vi "RT DAQ.vi"() -> ()   [LabVIEW 2023]
uses:
  <vilib>/rvi/interface/nirviOpenFPGA/nirviOpenFPGA.xnode
  <vilib>/rvi/interface/nirviMethod/nirviMethod.xnode
  <vilib>/FPGAPlugInAG/Dynamic/niLvFpga_Run_Dynamic.vi
  <vilib>/rvi/interface/nirviMethod/StockFPGA_InlinedMethodWaitForSingleIRQ.vi
  <vilib>/FPGAPlugInAG/Dynamic/niLvFpga_WaitOnIrq_Dynamic.vi
  <vilib>/FPGAPlugInAG/Dynamic/niLvFpga_AcknowledgeIrq_Dynamic.vi
  <vilib>/FPGAPlugInAG/Dynamic/niLvFpga_Reset_Dynamic.vi
  <vilib>/rvi/interface/nirviReadWriteControl/nirviReadWriteControl.xnode
  NiFpgaLv.dll
  <vilib>/Utility/error.llb/Error Cluster From Error Code.vi
  <vilib>/rvi/interface/Simulation/niFpgaSimulationCallBeginRW.vi
  <vilib>/rvi/errors/niLvFpgaAdjustHostInterfaceError.vi
  <vilib>/rvi/interface/nirviCloseFPGA/nirviCloseFPGA.xnode
  <vilib>/NI_Real-Time Target Support.lvlib
  <vilib>/FPGAPlugInAG/Dynamic/niLvFpga_Close_Dynamic.vi
  Transport measurement/FPGA Bitfiles/Mainproject_FPGATarget_SinglepointDAQ2_KFK63D1NkjA.lvbitx
  Single point DAQ.vi
  <vilib>/FPGAPlugInAG/cRIO-9063/niLvFpga_Open_cRIO-9063.vi
  <vilib>/rvi/interface/common/dynamic/niFpgaDynamicAddResources.vi
panel:
  out "VI Stop":bool
  out "error out":errorcluster
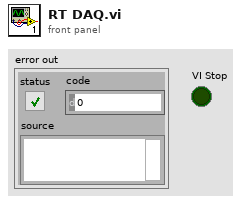
[diagram p1: front panel]
types:
  T1 = cluster{"Command":string, "Voltage":dbl, "Channel":string}
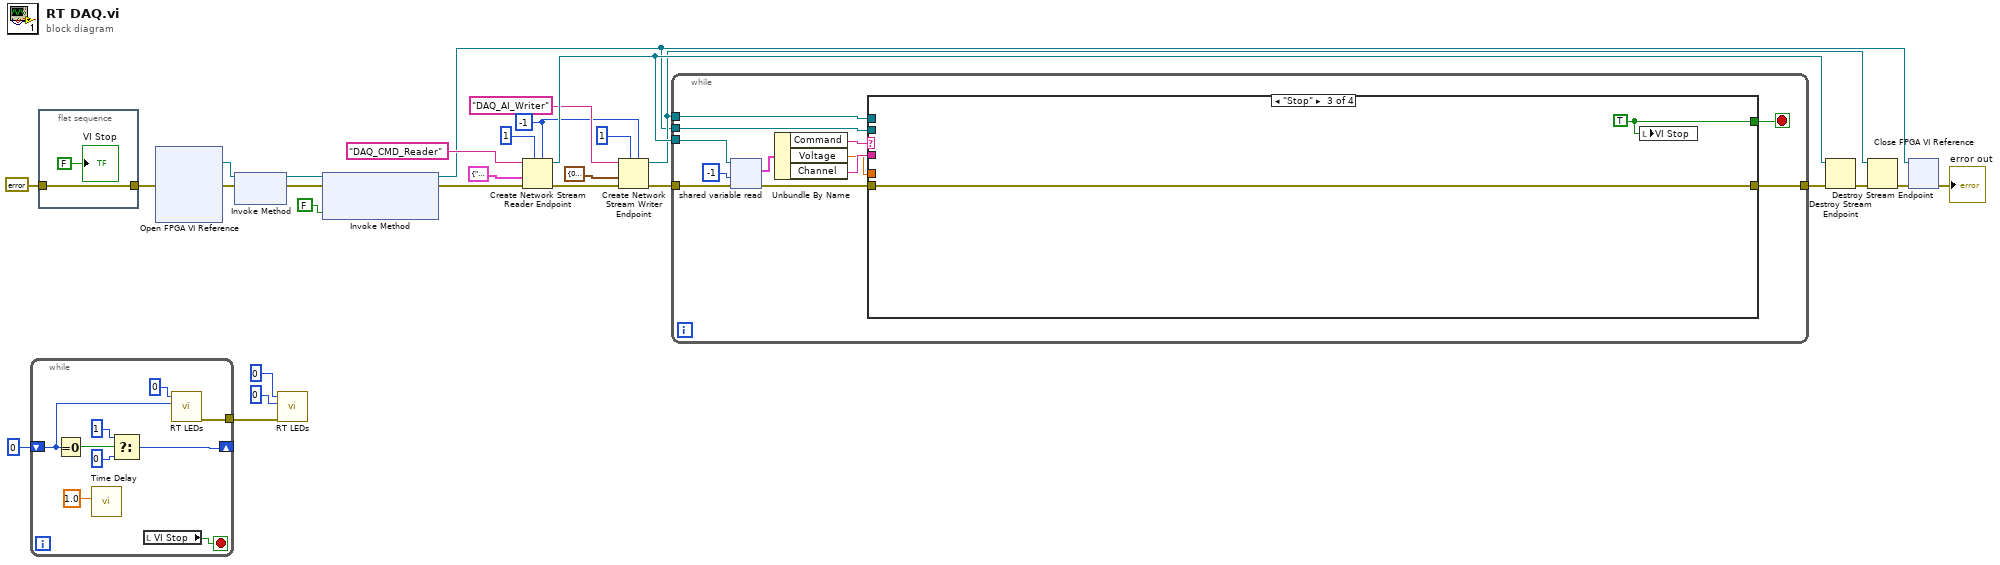
[diagram p0: block diagram]
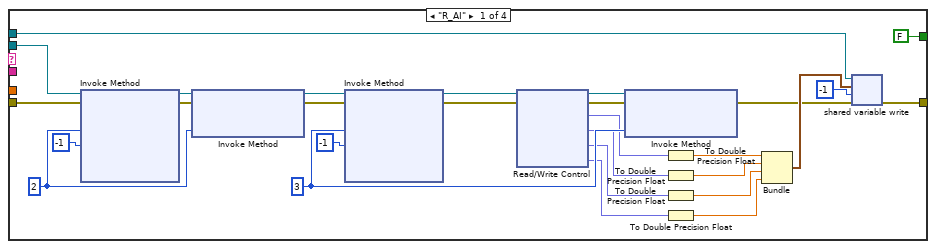
[diagram p2: hidden frame]
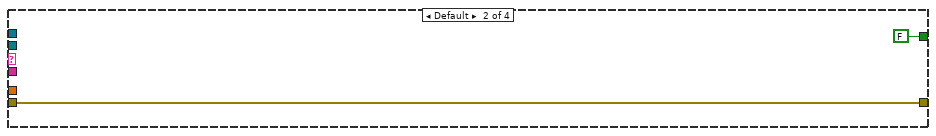
[diagram p3: hidden frame]
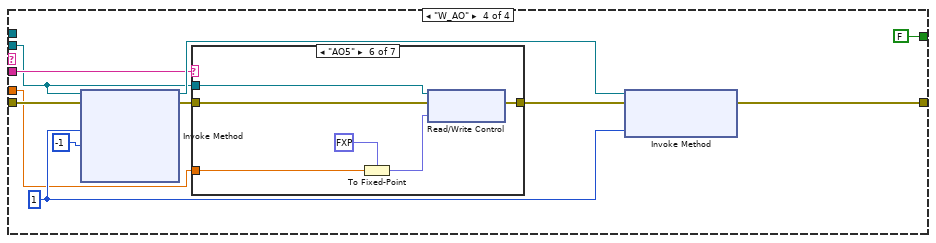
[diagram p4: hidden frame]
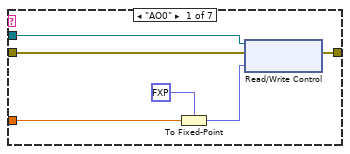
[diagram p5: hidden frame]
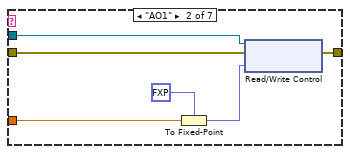
[diagram p6: hidden frame]
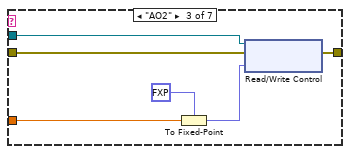
[diagram p7: hidden frame]
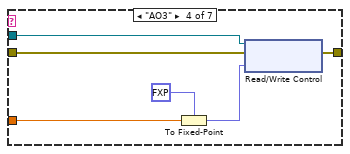
[diagram p8: hidden frame]
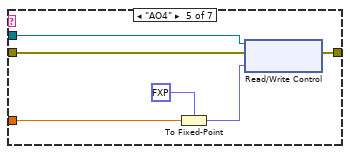
[diagram p9: hidden frame]
diagram:
  w1 = -1 ("timeout in ms (-1)")
  n1 = while {
    shift-right: [w32] -> _
    shift-left: 0 ("State") -> [w36]
    tunnel: [w29] -> w4
    stop <- w30 stop-if-true
    n2 = Equal To 0?(x=w36) -> (x = 0?=w35:bool)
    n3 = call "Time Delay"("Delay Time (s)"=1.0) -> ()  [unwired: 10 in, 1 out]
    n4 = Select(t=1, s=w35, f=0) -> (s? t:f=w32:i32)
    n5 = local read "VI Stop"() -> (w30:bool)
    n6 = call <vilib>:"RT LEDs.vi"("State"=w36, "LED Num"=0) -> ("error out"=w29:errorcluster)  [unwired: 4 in, 1 out]
  }
  n7 = flat-sequence {
    tunnel: errorcluster {"status"=FALSE, "code"=0, "source"=""} ("error in (no error)") -> [w39]
    tunnel: [w39] -> w2
    frame #0 {
      "VI Stop" <- FALSE ("VI Stop")
    }
  }
  n8 = xnode "Open FPGA VI Reference"("error in"=w2) -> ("FPGA VI Reference Out"=w24:refnum<k20>, "error out"=w23:errorcluster)  [unwired: 1 in]
  n9 = xnode "Invoke Method"("FPGA VI Reference In"=w24, "error in"=w23) -> ("FPGA VI Reference Out"=w25:refnum<k20>, "error out"=w22:errorcluster)
  n10 = call <vilib>:"RT LEDs.vi"("error in (no error)"=w4, "State"=0, "LED Num"=0) -> ()  [unwired: 3 in, 2 out]
  n11 = xnode "Invoke Method"("FPGA VI Reference In"=w25, "error in"=w22, "Wait Until Done (F)"=FALSE) -> ("FPGA VI Reference Out"=w11:refnum<k20>, "error out"=w17:errorcluster)
  n12 = Create Network Stream Reader Endpoint(5:w1, 7:1 ("reader buffer size"), 8:w17, 9:T1 {"Command"="", "Voltage"=0.0, "Channel"=""} ("Write cluster"), 11:"DAQ_CMD_Reader" ("reader name")) -> (0:w14:errorcluster, 3:w20:refnum<k21>)  [unwired: 2 in]
  n13 = Create Network Stream Writer Endpoint(5:w1, 7:1 ("writer buffer size"), 8:w14, 9:cluster{dbl, dbl, dbl, dbl} {0.0, 0.0, 0.0, 0.0} ("output cluster"), 11:"DAQ_AI_Writer" ("reader name")) -> (0:w9:errorcluster, 3:w13:refnum<k21>)  [unwired: 2 in]
  n14 = while {
    tunnel: w9 -> [w51]
    tunnel: w20 -> [w50]
    tunnel: w11 -> [w46]
    tunnel: [w41] -> w21
    tunnel: w13 -> [w42]
    stop <- w40 stop-if-true
    n15 = shared-variable-read(w50, w51, -1 ("timeout ms (-1)")) -> (w45:errorcluster, w48:T1)  [unwired: 2 out]
    n16 = Unbundle By Name(w48) -> ("Command"=w47:string, "Voltage"=w43:dbl, "Channel"=w44:string)
    n17 = case shown="\"Stop\"" w47 {
      tunnel: w46 -> [w74 _ _ w87]
      tunnel: w45 -> [w75 w80 w83 w90]
      tunnel: w44 -> [_ _ _ w88]
      tunnel: w43 -> [_ _ _ w86]
      tunnel: [w53 w80 w83 w85] -> w41
      tunnel: w42 -> [w65 _ _ _]
      tunnel: [FALSE FALSE w82 FALSE] -> w40
      frame "R_AI" {
        w73 = 3 ("IRQ Number(s)")
        w77 = 2 ("IRQ Number(s)")
        n18 = xnode "Invoke Method"("FPGA VI Reference In"=w74, "error in"=w75, "IRQ Number(s)"=w77, "Timeout (ms)"=-1) -> ("FPGA VI Reference Out"=w78:refnum<k20>, "error out"=w79:errorcluster)  [unwired: 2 out]
        n19 = xnode "Invoke Method"("FPGA VI Reference In"=w78, "error in"=w79, "IRQ Number(s)"=w77) -> ("FPGA VI Reference Out"=w71:refnum<k20>, "error out"=w70:errorcluster)
        n20 = xnode "Invoke Method"("FPGA VI Reference In"=w71, "error in"=w70, "IRQ Number(s)"=w73, "Timeout (ms)"=-1) -> ("FPGA VI Reference Out"=w69:refnum<k20>, "error out"=w68:errorcluster)  [unwired: 2 out]
        n21 = xnode "Read/Write Control"("FPGA VI Reference In"=w69, "error in"=w68) -> ("FPGA VI Reference Out"=w67:refnum<k20>, "error out"=w66:errorcluster, "Mod1/AI0"=w64:fxp<+/-,17,5>, "Mod1/AI1"=w63:fxp<+/-,17,5>, "Mod1/AI2"=w62:fxp<+/-,17,5>, "Mod1/AI3"=w61:fxp<+/-,17,5>)
        n22 = xnode "Invoke Method"("FPGA VI Reference In"=w67, "error in"=w66, "IRQ Number(s)"=w73) -> ("error out"=w55:errorcluster)  [unwired: 1 out]
        n23 = To Double Precision Float(number=w64) -> (double precision float=w60:dbl)
        n24 = To Double Precision Float(number=w63) -> (double precision float=w59:dbl)
        n25 = To Double Precision Float(number=w62) -> (double precision float=w58:dbl)
        n26 = To Double Precision Float(number=w61) -> (double precision float=w57:dbl)
        n27 = Bundle(w60, w59, w58, w57) -> (w56:cluster{dbl, dbl, dbl, dbl})  [unwired: 1 in]
        n28 = shared-variable-write(w65, w55, w56, -1 ("timeout ms (-1)")) -> (w53:errorcluster)  [unwired: 2 out]
      }
      frame Default {
      }
      frame "Stop" {
        w82 = TRUE
        n29 = local write "VI Stop"(w82) -> ()
      }
      frame "W_AO" {
        w91 = 1 ("IRQ Number(s)")
        n30 = xnode "Invoke Method"("FPGA VI Reference In"=w87, "error in"=w90, "IRQ Number(s)"=w91, "Timeout (ms)"=-1) -> ("FPGA VI Reference Out"=w92:refnum<k20>, "error out"=w93:errorcluster)  [unwired: 2 out]
        n31 = case shown="\"AO5\"" w88 {
          tunnel: w87 -> [w100 w104 w110 w116 w122 w128 _]
          tunnel: w86 -> [w97 w102 w109 w115 w120 w126 _]
          tunnel: w93 -> [w96 w103 w108 w114 w121 w127 w131]
          tunnel: [w95 w101 w107 w113 w119 w125 w131] -> w94
          frame "AO0" {
            n32 = To Fixed-Point(fixed-point type=fxp<+/-,20,5> 0.0 ("Mod3/AO0"), number=w97) -> (fixed-point=w98:fxp<+/-,20,5>)
            n33 = xnode "Read/Write Control"("FPGA VI Reference In"=w100, "error in"=w96, "Mod3/AO0"=w98) -> ("error out"=w95:errorcluster)  [unwired: 1 out]
          }
          frame "AO1" {
            n34 = To Fixed-Point(fixed-point type=fxp<+/-,20,5> 0.0 ("Mod3/AO0"), number=w102) -> (fixed-point=w105:fxp<+/-,20,5>)
            n35 = xnode "Read/Write Control"("FPGA VI Reference In"=w104, "error in"=w103, "Mod3/AO1"=w105) -> ("error out"=w101:errorcluster)  [unwired: 1 out]
          }
          frame "AO2" {
            n36 = To Fixed-Point(fixed-point type=fxp<+/-,20,5> 0.0 ("Mod3/AO0"), number=w109) -> (fixed-point=w111:fxp<+/-,20,5>)
            n37 = xnode "Read/Write Control"("FPGA VI Reference In"=w110, "error in"=w108, "Mod3/AO2"=w111) -> ("error out"=w107:errorcluster)  [unwired: 1 out]
          }
          frame "AO3" {
            n38 = To Fixed-Point(fixed-point type=fxp<+/-,20,5> 0.0 ("Mod3/AO0"), number=w115) -> (fixed-point=w117:fxp<+/-,20,5>)
            n39 = xnode "Read/Write Control"("FPGA VI Reference In"=w116, "error in"=w114, "Mod3/AO3"=w117) -> ("error out"=w113:errorcluster)  [unwired: 1 out]
          }
          frame "AO4" {
            n40 = To Fixed-Point(fixed-point type=fxp<+/-,20,5> 0.0 ("Mod3/AO0"), number=w120) -> (fixed-point=w123:fxp<+/-,20,5>)
            n41 = xnode "Read/Write Control"("FPGA VI Reference In"=w122, "error in"=w121, "Mod3/AO4"=w123) -> ("error out"=w119:errorcluster)  [unwired: 1 out]
          }
          frame "AO5" {
            n42 = To Fixed-Point(fixed-point type=fxp<+/-,20,5> 0.0 ("Mod3/AO0"), number=w126) -> (fixed-point=w129:fxp<+/-,20,5>)
            n43 = xnode "Read/Write Control"("FPGA VI Reference In"=w128, "error in"=w127, "Mod3/AO5"=w129) -> ("error out"=w125:errorcluster)  [unwired: 1 out]
          }
          frame Default {
          }
        }
        n44 = xnode "Invoke Method"("FPGA VI Reference In"=w92, "error in"=w94, "IRQ Number(s)"=w91) -> ("error out"=w85:errorcluster)  [unwired: 1 out]
      }
    }
  }
  n45 = Destroy Stream Endpoint(8:w21, 11:w20) -> (0:w19:errorcluster)
  n46 = Destroy Stream Endpoint(8:w19, 11:w13) -> (0:w10:errorcluster)
  n47 = xnode "Close FPGA VI Reference"("FPGA VI Reference In"=w11, "error in"=w10) -> ("error out"=→"error out":errorcluster)
